vi "Pre Launch Init.vi"(11 "Nested in":refnum<class "Prooduct Actor.lvclass">) -> (0 "error out":errorcluster, 3 "Nested out":refnum<class "Prooduct Actor.lvclass">)   [LabVIEW 2020, in "Prooduct Actor.lvlib" / "Prooduct Actor.lvclass"]
doc: "(<B>Filename</B>: Actor Framework.lvlib:Actor.lvclass:Pre Launch Init.vi)\n\nDefines behavior that occurs after the Launch Nested Actor method is invoked but before the actor's Actor Core method begins running.\n\nBy default, this method does nothing. A descendant class may override it to define behavior."
uses:
  Prooduct Actor.lvclass
  C:/Program Files (x86)/National Instruments/LabVIEW 2020/vi.lib/ActorFramework/Actor/Actor.lvclass
  Controls/Language Enum.ctl
  Controls/Currency Enum.ctl
  Prooduct Actor.lvclass/Prooduct Actor.ctl
  <vilib>/ActorFramework/Actor/Actor.lvclass/Actor.ctl
  <vilib>/ActorFramework/Message Enqueuer/Message Enqueuer.lvclass/Message Enqueuer.ctl
  <vilib>/ActorFramework/Message Enqueuer/Enqueue.vi
  <vilib>/ActorFramework/Message Enqueuer/Init from Existing Queue.vi
  Prooduct Actor Messages/Initialization Msg/Initialization Msg.lvclass
  C:/Program Files (x86)/National Instruments/LabVIEW 2020/vi.lib/ActorFramework/Message/Message.lvclass
  Prooduct Actor Messages/ButtonLanguage Msg/ButtonLanguage Msg.lvclass
  Prooduct Actor Messages/UpdateList Msg/UpdateList Msg.lvclass
  <vilib>/ActorFramework/Message Priority Queue/Priority Enqueue.vi
  <vilib>/ActorFramework/Message Enqueuer/Message Enqueuer.lvclass
  <vilib>/ActorFramework/Actor/Actor.lvclass
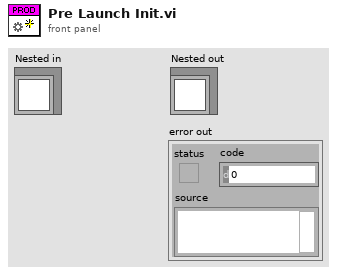
[diagram p1: front panel]
types:
  T1 = typedef "Language Enum.ctl" = enum16{"English", "Español", "Français"}
  T2 = typedef "Currency Enum.ctl" = enum16{"USD", "MXN", "EUR"}
  T3 = cluster{"Language":T1, "Currency":T2, "DB Path":path}
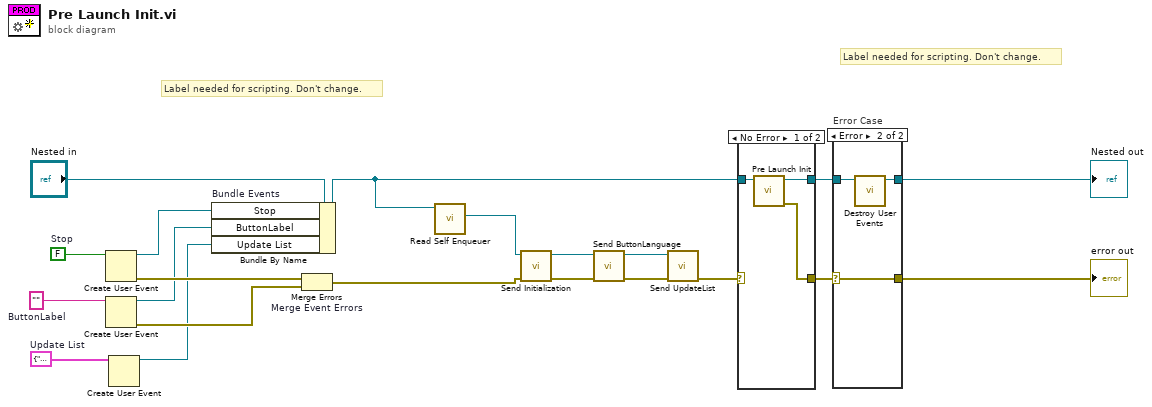
[diagram p0: block diagram]
diagram:
  w5 = T3 {"Language"=enum."English", "Currency"=enum."USD", "DB Path"=path ""}  # Update List
  w12 = ""  # ButtonLabel
  w20 = FALSE  # Stop
  # "Label needed for scripting. Don't change."
  # "Label needed for scripting. Don't change."
  n1 = Create User Event(user event datatype=w20) -> (user event=w17:refnum<user-event>, error out=w19:errorcluster)  [unwired: 1 in]
  n2 = Create User Event(user event datatype=w12) -> (user event=w11:refnum<user-event>, error out=w13:errorcluster)  [unwired: 1 in]
  n3 = Create User Event(user event datatype=w5) -> (user event=w4:refnum<user-event>)  [unwired: 1 in, 1 out]
  n4 = Bundle By Name "Bundle Events"(cluster="Nested in", "Stop"=w17, "ButtonLabel"=w11, "Update List"=w4) -> (w10:refnum<class "Prooduct Actor.lvclass">)
  n5 = Merge Errors "Merge Event Errors"(w19, w13) -> (w6:errorcluster)
  n6 = call <vilib>:"Read Self Enqueuer.vi"("Actor"=w10) -> ("Self Enqueuer"=w7:refnum<class "Message Enqueuer.lvclass">)  [unwired: 10 in]
  n7 = call "Send Initialization.vi"("error in (no error)"=w6, "Message Enqueuer"=w7) -> ("error out"=w9:errorcluster, "Message Enqueuer out"=w8:refnum<class "Message Enqueuer.lvclass">)  [unwired: 8 in]
  n8 = call "Send ButtonLanguage.vi"("error in (no error)"=w9, "Message Enqueuer"=w8) -> ("error out"=w3:errorcluster, "Message Enqueuer out"=w1:refnum<class "Message Enqueuer.lvclass">)  [unwired: 8 in]
  n9 = call "Send UpdateList.vi"("error in (no error)"=w3, "Message Enqueuer"=w1) -> ("error out"=w2:errorcluster)  [unwired: 8 in, 1 out]
  n10 = case shown="No Error" w2 {
    selector: w2 -> [_ w26]
    tunnel: [w24 w25] -> w15
    tunnel: w10 -> [w23 w25]
    tunnel: [w22 w26] -> w14
    frame No Error {
      n11 = call-parent "Pre Launch Init.vi"("Actor in"=w23) -> ("error out"=w22:errorcluster, "Actor out"=w24:refnum<class "Prooduct Actor.lvclass">)  [unwired: 9 in]
    }
    frame Error {
    }
  }
  n12 = case "Error Case" shown="Error" w14 {
    selector: w14 -> [w27 w31]
    tunnel: w15 -> [w28 w30]
    tunnel: [w28 w29] -> w18
    tunnel: [w27 w31] -> w16
    frame No Error {
    }
    frame Error {
      n13 = call "Destroy User Events.vi"("UI Template in"=w30) -> ("UI Template out"=w29:refnum<class "Prooduct Actor.lvclass">)  [unwired: 10 in]
    }
  }
  "error out" <- w16
  "Nested out" <- w18
